vi "Periodic Tasks.vi"(8 "error in":errorcluster) -> ()   [LabVIEW 2014]
doc: "This VI runs in parallel to other tasks. It can contain as many user-defined periodic loops as you need. These can carry out PID or other sorts of timed response."
uses:
  1756_Code/General_VI/Global Var.vi
  <vilib>/Rock Robotics/Network Tables/SD Write Numeric Array.vi
panel:
  out "output cluster":T1
  in  "Num_Avg":dbl=10.0
  out "Autro":T2
  out "Master_Auto_Stop_Value":bool
  out "Auto_State":dbl(graph)
  in  "Reset_Enable":bool
  out "Compressor Running":bool
  out "Compressor Monitoring":bool
  out "Yaw":dbl
  out "Yaw":cluster{dbl, dbl}(knob)={0.0, 152.0639793131716} scale=-180.0..180.0
  out "Z Ang":dbl(graph)
  out "FreeFall":bool
  out "Motion":bool
  out "Anomaly":bool
  out "R/P Alpha":dbl
  out "Yaw Alpha":dbl
  in  "tau acc (s)":dbl=0.047 format="%#_13g"
  in  "tau mag (s)":dbl=0.06 format="%#_13g"
  in  "Tilt Comp (Yaw)":bool
  # "FRC Team 836, The RoboBees: Sensor Fusion Demonstration / Designed for roboRIO\nDescription:\nThis series of Inertial Measurement Unit (IMU) subVIs is patterened after the WPI series for reading sensors, and includes several\nadditional IMU Application subVIs.  These application subVIs do the math required for sensor fusion, forming a basic Attitude\nand Heading Reference System (AHRS), with drift-free Roll, Pitch and Yaw outputs.  An IMU typically consists of a 3-axis \nAccelerometer, Rate Gyroscope, and Magnetometer (sometimes the Mag is absent, resulting in reduced capability).  Although\ntechnically incorrect, these devices are often referred to as 9 Degrees-of-Freedom (DoF) sensors (3 sensors with each 3\naxes in XYZ = 9 DoF). \n\nCompatible IMUs:\nThese IMU subVIs are designed to be used with the Adafruit 9-DoF IMU Breakout - containing L3GD20 (Gyro) + LSM303 \n(Accelerometer and Magnetometer) chips (Product ID: 1714), or the Adafruit 10-DoF IMU Breakout - whichs adds the BMP180\nchip (Product ID: 1604).  The 10-DoF IMU adds a Barometer for air temperature and pressure measurements (for indicating\naltitude, not attitude), and is not currently implemented.  The two IMU Application subVIs, COMPLE FILTER and TILT, are\nagnostic of IMU model, and compatible with separate sensors, as long as all sensor axes are aligned properly."
  # "AdaFruit 1714"
  # "Sensor Orientation:\nWhen Sensor oriented with positive X-axis\npointing forward, and positive Y-axis\npointing left, and positive Z axis pointing up :\n\nRoll is rotation about X-axis, clockwise roll,\n(looking in + X direction), is positive.\n\nPitch is rotation about Y-axis, clockwise pitch\n(looking in + Y direction), is positive.\n\nYaw is rotation about Z-axis, clockwise yaw\n(looking in + Z direction), is positive."
  # "Robot\nFront"
  # "RoboBees IMU and AHRS Demo Instructions:\n(1) Connect IMU to I2C port (4 wires: 5v/Gnd/SDA/SCK) on roboRIO.\n      Secure the IMU on Robot, orient as described at right.\n(2) Change the IP address of the roboRIO in the RoboBees IMU Demo project.\nYou can do this by right-clicking on RT CompactRIO Target in the project, selecting\nProperties, and modifying the IP Address setting in the General Category to match\nthat of your roboRIO.\n(3) Open Front Panel of the IMU OPEN subVI, you'll need that for step 8.\n(4) Establish Comm and Run this program (use Run Button deploy, not Build and deploy).\n(5) Follow the dialog boxes to perform Magnetometer Calibration.\n(6) Upon cal completion, observe Roll, Pitch, Yaw gauges as you (re)orient your sensor/robot.\n(7) Observe the 9 DoF display graphs for Gyro, Accel, and Mag in each XYZ axes.  The graphs are\n       useful in understanding how the sensors respond, but it's best to disable them once you no\n       longer need them, as they slow the dynamic response of the code under a Run button\n       deploy.  A simple way to do this is to wrap a Diagram Disable Structure (Structures Menu)\n       around the chart indicators on the Block Diagram. \n(8) Observe result of Magnetometer cal graph on the IMU OPEN front panel.  Use adjacent\n      graph display for reference.\n(9) If you don't like Mag cal result, repeat Mag cal by rerunning program.  See comments\nin IMU OPEN code for guidance.  If cal ok, stop program and load the 4 Mag cal\nparameters displayed in IMU OPEN (two each for X and Y axes), into Mag Set Cluster just below.\n(10) Set MagCal switch to false, then rerun this program.  This config is for competition.\n(11) Adjust the Loop Period as desired.  See implementation notes in IMU READ VI for guidance.\n(12) Adjust the Accelerometer tau and Magnetometer tau values as desired.  See implementation\n       notes in COMPLE FILTER VI  for guidance.\n(13) The Gyro/Accel cal process w/in IMU OPEN will auto-recal if it detects excessive\n        variation in the sample dataset, which likely indicates robot was bumped during cal.\n        Gently shake robot during program startup and observe BadCal indicators.\n(14) The roboRIO has two seperate I2C buses, On-Board and MXP.  This code works with the\n        On-Board I2C bus, but currently throws an error on the MXP I2C bus, tested with a Rev\n        Robotics expansion board.  \n\nPls provide attribution to FRC Team 836, The RoboBees if you find this useful !!"
  # "roboRIO I2C    DIO-0  V     Gnd    SCL     SDA"
  # "Sensor Fusion Design:"
  # "Note that Period (dt) can probably be reduced to less than 20 ms before Timed Loop starts running late, in this demo, since it's the only code running.  Using these IMU VIs in your code, however, may require a longer loop period to allow the CPU time to execute your other robot code  - you can use the same technique of adjusting the period while monitoring the Late indicator for optimization when you integrate these VIs into your code.  You can disable the 9 DoF graphs to considerably improve speed of code (when deployed with the Run button), in which case Period can be much lower (~3 ms, again, provided this is the only code running).  Benchmark was against 2015 roboRIO."
  # "Sensor Fusion Settings"
  # "Adjust these tau settings to optimize the sensor fusion.  tau acc affects\nRoll and Pitch.  tau mag affects Yaw.   Consider that alpha = tau / (tau + dt),\nand that alpha is what affects the fusion performance.  An alpha of about 0.7 for\nRoll and Pitch, and an alpha of about 0.6 for Yaw appear to be good starting points."
  # "Enabling this corrects Yaw error when Pitch and Roll are\nnon-zero, however, Yaw will be affected by Accelerometer\nmovement and noise.  Reference IMU Comple Filter subVI\nnotes for more insight on this tradeoff."
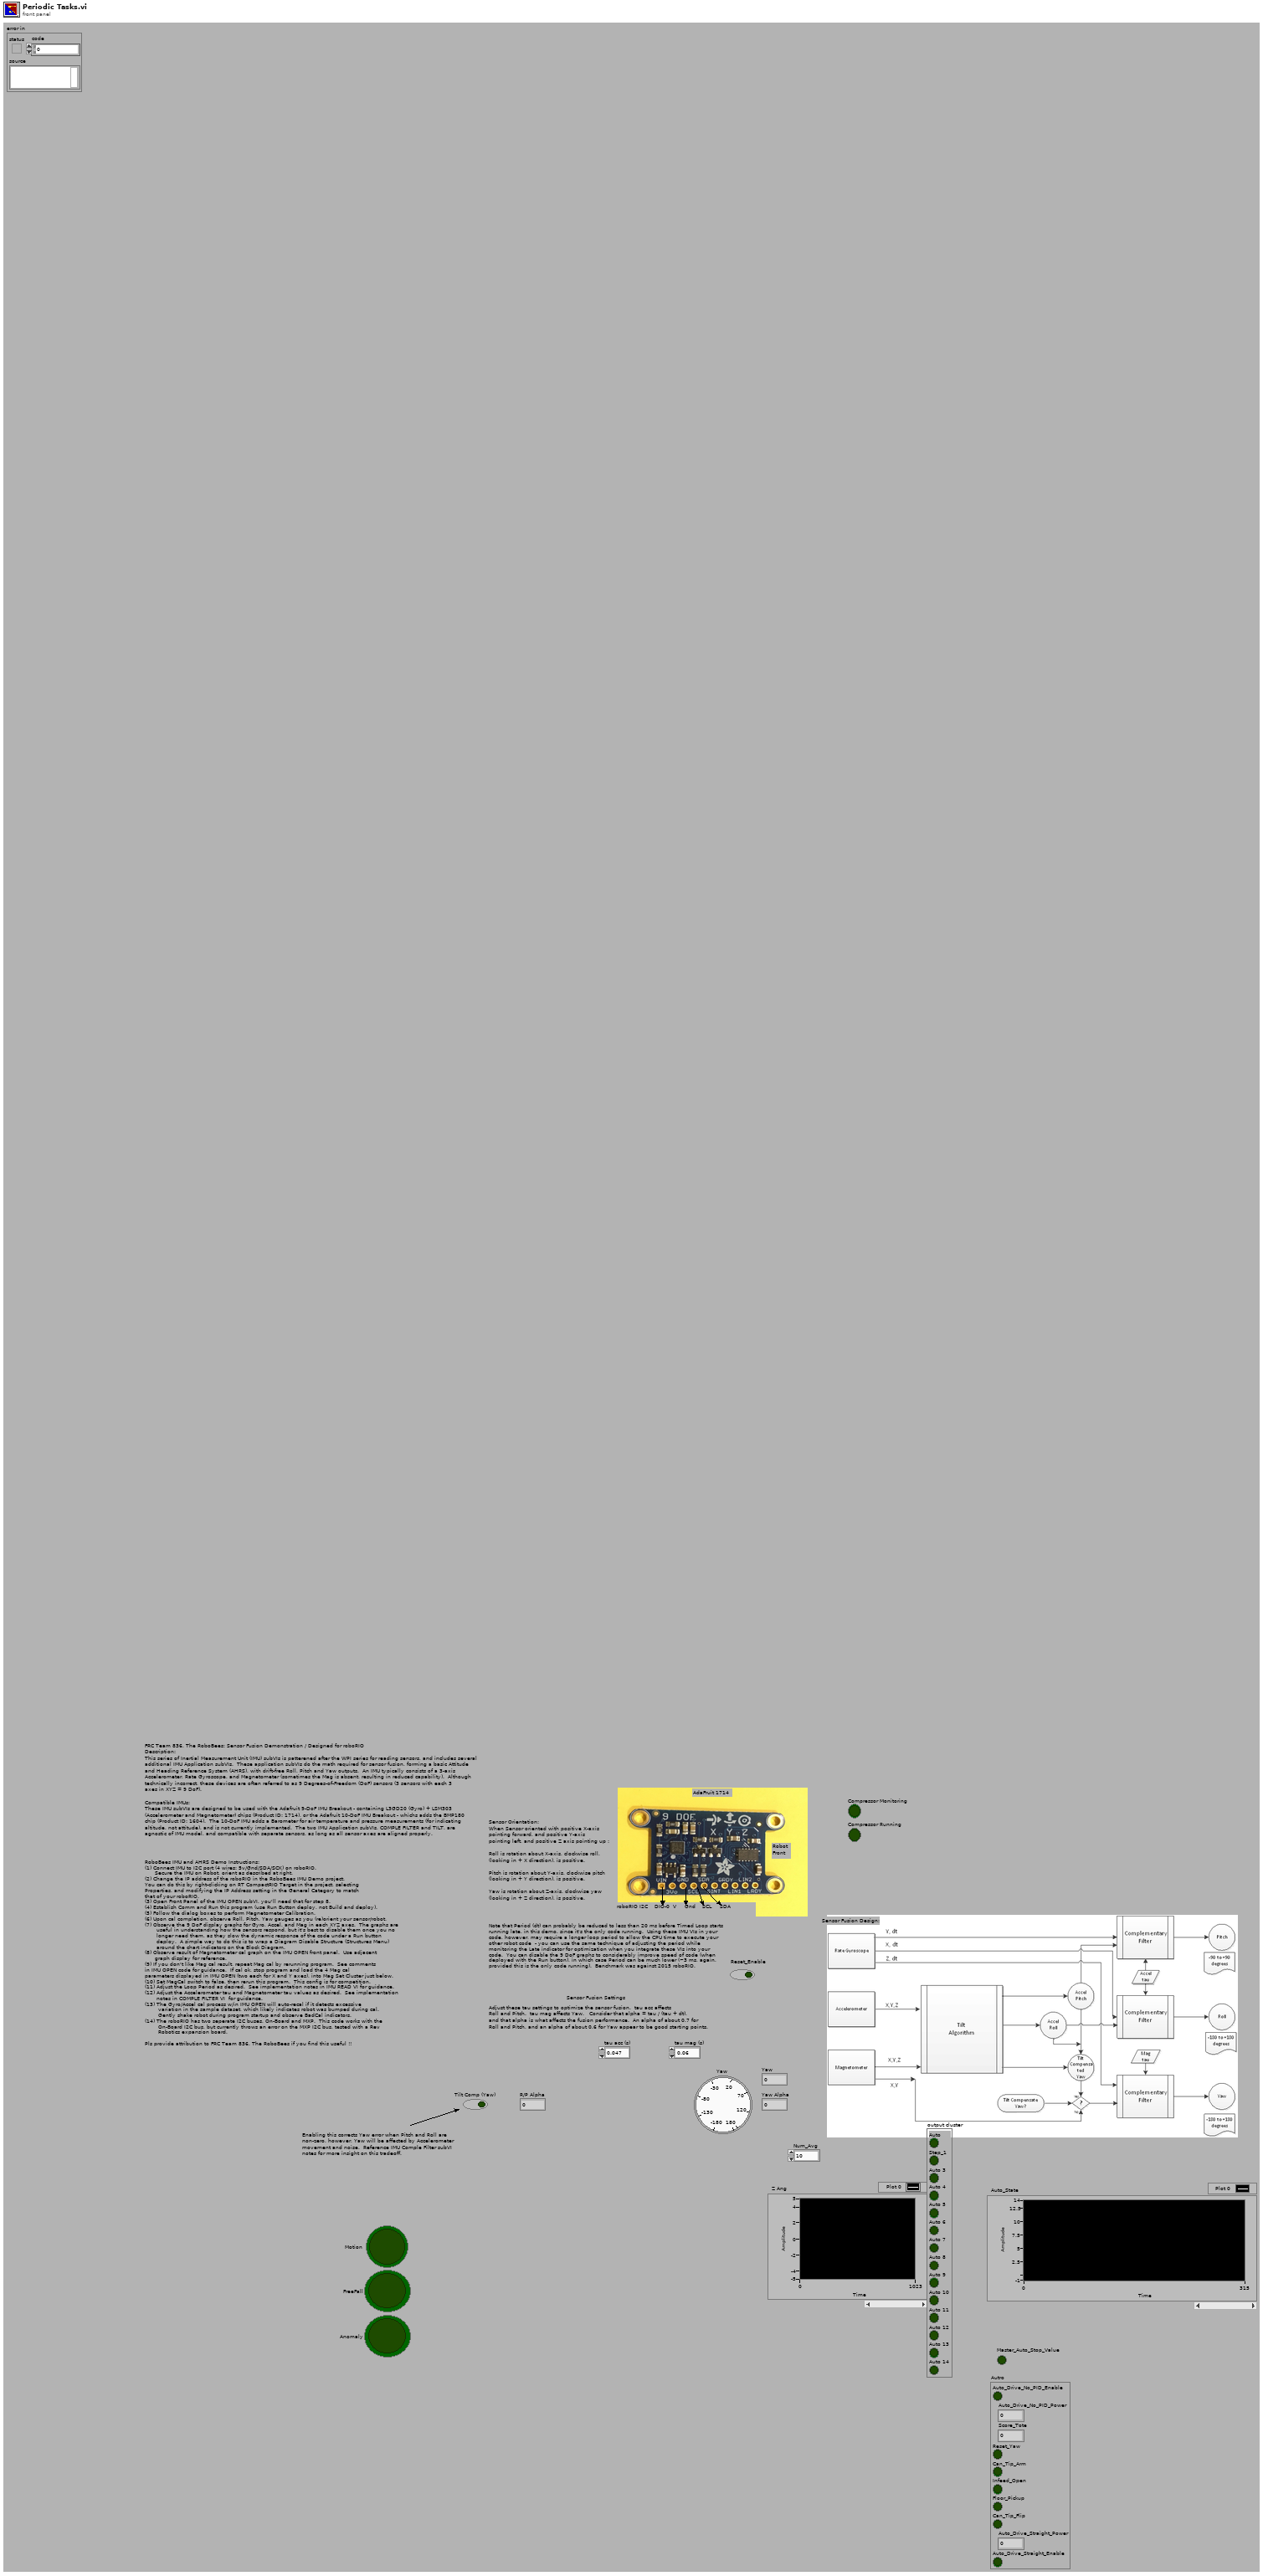
[diagram p1: front panel]
types:
  T1 = cluster{"Auto":bool, "Step_1":bool, "Auto 3":bool, "Auto 4":bool, "Auto 5":bool, "Auto 6":bool, "Auto 7":bool, "Auto 8":bool, "Auto 9":bool, "Auto 10":bool, "Auto 11":bool, "Auto 12":bool, "Auto 13":bool, "Auto 14":bool}
  T2 = cluster{"Auto_Drive_No_PID_Enable":bool, "Auto_Drive_No_PID_Power":dbl, "Score_Tote":dbl, "Reset_Yaw":bool, "Can_Tip_Arm":bool, "Infeed_Open":bool, "Floor_Pickup":bool, "Can_Tip_Flip":bool, "Auto_Drive_Straight_Power":dbl, "Auto_Drive_Straight_Enable":bool}
  T3 = typedef "WPI_JoystickDevRef.ctl" = cluster{"Device":T4}
  T4 = typedef "WPI_JoystickDeviceEnum.ctl" = enum16{"USB 0", "USB 1", "USB 2", "USB 3", "USB 4", "USB 5"}
  T5 = typedef "WPI_RobotDriveDevRef.ctl" = cluster{"DevStatus":errorcluster, "Motors[]":T6[], "Square Inputs":bool, "Max Output":dbl}
  T6 = typedef "WPI_MotorControlDeviceRef.ctl" = cluster{"DeviceStatus":errorcluster, "Type":T7, "PWM":cluster{"Controller":T8, "PWM Channel":T9, "DeadBand":T10}, "CAN":cluster{"Device Number":u8, "Control Mode":T11, "Semaphore":T12, "Max Vout":dbl, "TalonSRX Control Mode":T13}, "Invert":bool, "TransformRef":T14, "InvTransformRef":T14}
  T7 = typedef "WPI_MotorControlType.ctl" = enum16{"PWM", "CAN", "CANTalonSRX"}
  T8 = typedef "FPGA_TypedefDigitalModule.ctl" = enum16{"Controller 1"}
  T9 = typedef "FPGA_DIOPWMChannel.ctl" = enum8{"PWM 0", "PWM 1", "PWM 2", "PWM 3", "PWM 4", "PWM 5", "PWM 6", "PWM 7", "PWM 8", "PWM 9", "PWM MXP 0", "PWM MXP 1", "PWM MXP 2", "PWM MXP 3", "PWM MXP 4", "PWM MXP 5", "PWM MXP 6", "PWM MXP 7", "PWM MXP 8", "PWM MXP 9", "Invalid"}
  T10 = typedef "WPI_PWMDeadband.ctl" = cluster{"Name":string, "maxPositivePwm":i32, "minPositivePwm":i32, "centerPwm":i32, "maxNegativePwm":i32, "minNegativePwm":i32, "angularRange":u16}
  T11 = typedef "WPI_CANJaguar_ControlMode.ctl" = enum8{"Percent VBus", "Current", "Speed", "Position", "Voltage"}
  T12 = typedef "Semaphore RefNum" = refnum<k1>
  T13 = typedef "WPI_CANTalonSRX_APIControlMode.ctl" = enum8{"Percent VBus", "Speed", "Position", "Slave", "Unchanged / Invalid"}
  T14 = typedef "WPI_PWMTransform_ConPane.ctl" = refnum<vi>
  T15 = typedef "WPI_EncoderDevRef.ctl" = cluster{"DevStatus":errorcluster, "EncoderIndex":T16, "CounterIndex":T17, "DistancePerCount":dbl, "Decoding Type":T18}
  T16 = typedef "FPGA_EncoderIdx.ctl" = enum8{"Enc 0", "Enc 1", "Enc 2", "Enc 3", "Enc 4", "Enc 5", "Enc 6", "Enc 7", "Invalid"}
  T17 = typedef "FPGA_CounterCtrSystemIndex.ctl" = enum8{"Ctr 0", "Ctr 1", "Ctr 2", "Ctr 3", "Ctr 4", "Ctr 5", "Ctr 6", "Ctr 7", "Invalid"}
  T18 = typedef "WPI_EncoderType.ctl" = enum16{"1x", "2x", "4x"}
  T19 = typedef "WPI_SwitchDevRef.ctl" = cluster{"DevStatus":errorcluster, "DIO Channel":T20, "Controller":T8, "CntIndex":T17, "Normally Closed":bool}
  T20 = typedef "FPGA_DIOChannel.ctl" = enum8{"DIO 0", "DIO 1", "DIO 2", "DIO 3", "DIO 4", "DIO 5", "DIO 6", "DIO 7", "DIO 8", "DIO 9", "DIO MXP 0", "DIO MXP 1", "DIO MXP 2", "DIO MXP 3", "DIO MXP 4", "DIO MXP 5", "DIO MXP 6", "DIO MXP 7", "DIO MXP 8", "DIO MXP 9", "DIO MXP 10", "DIO MXP 11", "DIO MXP 12", "DIO MXP 13", "DIO MXP 14", "DIO MXP 15", "Invalid"}
  T21 = typedef "WPI_AnalogChannelDevRef.ctl" = cluster{"DevStatus":errorcluster, "Controller":T22, "Analog Channel":T23}
  T22 = typedef "FPGA_TypedefAnalogModule.ctl" = enum16{"Controller 1"}
  T23 = typedef "FPGA_AIChannel.ctl" = enum8{"AI 0", "AI 1", "AI 2", "AI 3", "AI MXP 0", "AI MXP 1", "AI MXP 2", "AI MXP 3", "Invalid"}
  T24 = typedef "IMUDevRef.ctl" = cluster{"DevStatus":errorcluster, "Gyro Address":u8, "Gyro Range":u8, "Mean Rates":cluster{"Xmo":dbl, "Ymo":dbl, "Zmo":dbl}, "StdDev Rates":cluster{"Xsdo":dbl, "Ysdo":dbl, "Zsdo":dbl}, "Fast":bool, "Reset":bool, "Accel Address":u8, "Accel Range":u8, "Accel Scale":cluster{"Xscale":dbl, "Yscale":dbl, "Zscale":dbl}, "Mag Address":u8, "Mag Range":u8, "G Sense":bool, "A Sense":bool, "M Sense":bool, "Accel Offset":cluster{"Xzero":dbl, "Yzero":dbl, "Zzero":dbl}, "Motion Thresh":dbl, "Mag Scale":cluster{"Xscale":dbl, "Yscale":dbl, "Zscale":dbl}, "Mag Offset":cluster{"Xzero":dbl, "Yzero":dbl, "Zzero":dbl}, "I2C Bus":T25, "Handle":i32, "Controller":T8, "Anomaly Thresh":dbl, "Local Mag":dbl}
  T25 = typedef "i2c_bus.ctl" = enum16{"I2C On-Board", "I2C MXP", "Invalid"}
  T26 = typedef "WPI_CompressorDevRef.ctl" = cluster{"DevStatus":errorcluster, "Pneumatics Control Module":u8}
  T27 = typedef "WPI_SolenoidDevRef.ctl" = cluster{"DevStatus":errorcluster, "Pneumatics Control Module":u8, "Forward Solenoid Channel":T28, "Reverse Solenoid Channel":T28}
  T28 = typedef "WPI_SolenoidChannel.ctl" = enum8{"Solenoid 0", "Solenoid 1", "Solenoid 2", "Solenoid 3", "Solenoid 4", "Solenoid 5", "Solenoid 6", "Solenoid 7", "Invalid"}
  T29 = cluster{"Joystick":cluster{"Drive_Joystick":T3, "Imp_Joystick":T3}, "Motor":cluster{"Left and Right Motors":T5, "Left_Intake":T6, "Right_Intake":T6, "Elevator_Lift":T6, "Elevator_Arm_Left":T6, "Elevator_Arm_Right":T6}, "Encoder":cluster{"Left_Drive_Speed":T15, "Auto_2_Tote":T19, "Auto_Cans":T19, "Auto_Cans_Delay":T19}, "Analog":cluster{"Tote_Detect_1":T21, "Tote_Detect_2":T21, "Ele_Pos_Yoyo":T21, "Auto_Switch":T21}, "IMU_Reft_Num":T24, "Pneumatics":cluster{"Compressor":T26, "Arm_Sol":T27, "Infeed_Pneu":T27, "Can_Tip_Flip":T27, "Can_Tip_Arm":T27, "Can_Door_Arm":T27, "Arm_Sol_Ext":T27}}
  T30 = cluster{"Store_Auto":bool, "Exit_Auto":bool, "Infeed cmd":dbl, "Store_Auto_High":bool}
  T31 = cluster{"Station_Auto":bool, "Pickup_2_Auto":bool, "Infeed_cmd":dbl, "Open_Infeed":bool}
  T32 = cluster{"Open_Infeed":bool, " Raise_to_Step":bool, "Step 1":bool, "Step_3":bool}
  T33 = cluster{"Global_Var":cluster{"Eject":dbl, "Eject_Manual":dbl, " Station_Pickup":bool, "Arm_Pos":bool, "Elevator":dbl, "Exit_Pos":bool, "Floor_Pickup":bool, "Reset_Yaw":bool, "Step_Pos":bool, "Store_Pos":bool, "Yaw":dbl, "Score_Tote":bool, "Score_Step":bool, "Carry":bool, "Step_3":bool, "Infeed_Open":bool, "Can_Tip_Arm":bool, "Can_Tip_Flip":bool, "Step_1":bool, "Can_Door":bool, "Store_High":bool}, "Sensor_Val":cluster{"Left_Drive_Distance":dbl, "Tote_Detect_1":bool, "Tote_Detect_2":bool, "Ele_Pos_Yoyo":dbl, "Ele_At_Pos in":bool}}
  T34 = cluster{"Eject":dbl, "Eject_Manual":dbl, " Station_Pickup":bool, "Arm_Pos":bool, "Elevator":dbl, "Exit_Pos":bool, "Floor_Pickup":bool, "Reset_Yaw":bool, "Step_Pos":bool, "Store_Pos":bool, "Yaw":dbl, "Score_Tote":bool, "Score_Step":bool, "Carry":bool, "Step_3":bool, "Infeed_Open":bool, "Can_Tip_Arm":bool, "Can_Tip_Flip":bool, "Step_1":bool, "Can_Door":bool, "Store_High":bool}
  T35 = cluster{"Left_Drive_Distance":dbl, "Tote_Detect_1":bool, "Tote_Detect_2":bool, "Ele_Pos_Yoyo":dbl, "Ele_At_Pos in":bool}
  T36 = cluster{"Global_Var":cluster{"Eject":dbl, "Eject_Manual":dbl, " Station_Pickup":bool, "Arm_Pos":bool, "Elevator":dbl, "Exit_Pos":bool, "Floor_Pickup":bool, "Reset_Yaw":bool, "Step_Pos":bool, "Store_Pos":bool, "Yaw":dbl, "Score_Tote":bool, "Score_Step":bool, "Carry":bool, "Step_3":bool, "Infeed_Open":bool, "Can_Tip_Arm":bool, "Can_Tip_Flip":bool, "Step_1":bool, "Can_Door":bool, "Store_High":bool}, "Sensor_Val":cluster{"Left_Drive_Distance":dbl, "Tote_Detect_1":bool, "Tote_Detect_2":bool, "Ele_Pos_Yoyo":dbl, "Ele_At_Pos in":bool}, "Floor":cluster{"Store_Auto":bool, "Exit_Auto":bool, "Infeed cmd":dbl, "Store_Auto_High":bool}, "Station":cluster{"Station_Auto":bool, "Pickup_2_Auto":bool, "Infeed_cmd":dbl, "Open_Infeed":bool}, "Score_Tote":cluster{"Lower to Exit":bool, "Open Arms":bool}, "Score_Step":cluster{"Open_Infeed":bool, " Raise_to_Step":bool, "Step 1":bool, "Step_3":bool}, "Carry_Auto":cluster{"Lower to Carry":bool, "Open Arms":bool}}
  T37 = cluster{"Global_Var":cluster{"Eject":dbl, "Eject_Manual":dbl, " Station_Pickup":bool, "Arm_Pos":bool, "Elevator":dbl, "Exit_Pos":bool, "Floor_Pickup":bool, "Reset_Yaw":bool, "Step_Pos":bool, "Store_Pos":bool, "Yaw":dbl, "Score_Tote":bool, "Score_Step":bool, "Carry":bool, "Step_3":bool, "Infeed_Open":bool, "Can_Tip_Arm":bool, "Can_Tip_Flip":bool, "Step_1":bool, "Can_Door":bool, "Store_High":bool}, "Sensor_Val":cluster{"Left_Drive_Distance":dbl, "Tote_Detect_1":bool, "Tote_Detect_2":bool, "Ele_Pos_Yoyo":dbl, "Ele_At_Pos in":bool}, "Floor":cluster{"Store_Auto":bool, "Exit_Auto":bool, "Infeed cmd":dbl, "Store_Auto_High":bool}, "Station":cluster{"Station_Auto":bool, "Pickup_2_Auto":bool, "Infeed_cmd":dbl, "Open_Infeed":bool}, "Score_Tote":cluster{"Lower to Exit":bool, "Open Arms":bool}, "Score_Step":cluster{"Open_Infeed":bool, " Raise_to_Step":bool, "Step 1":bool, "Step_3":bool}, "Carry_Auto":cluster{"Lower to Carry":bool, "Open Arms":bool}, "Pos_Arb":cluster{"Pos_Des":dbl, "Pos_Active":bool}}
  T38 = typedef "Gyro.ctl" = cluster{"Xrate":dbl, "Yrate":dbl, "Zrate":dbl, "Xdeg":dbl, "Ydeg":dbl, "Zdeg":dbl, "dt":dbl}
  T39 = typedef "Accel.ctl" = cluster{"Xaccel":dbl, "Yaccel":dbl, "Zaccel":dbl, "Motion":bool, "Threshold":dbl, "FreeFall":bool}
  T40 = typedef "Mag.ctl" = cluster{"Xmag":dbl, "Ymag":dbl, "Zmag":dbl, "Anomaly":bool}
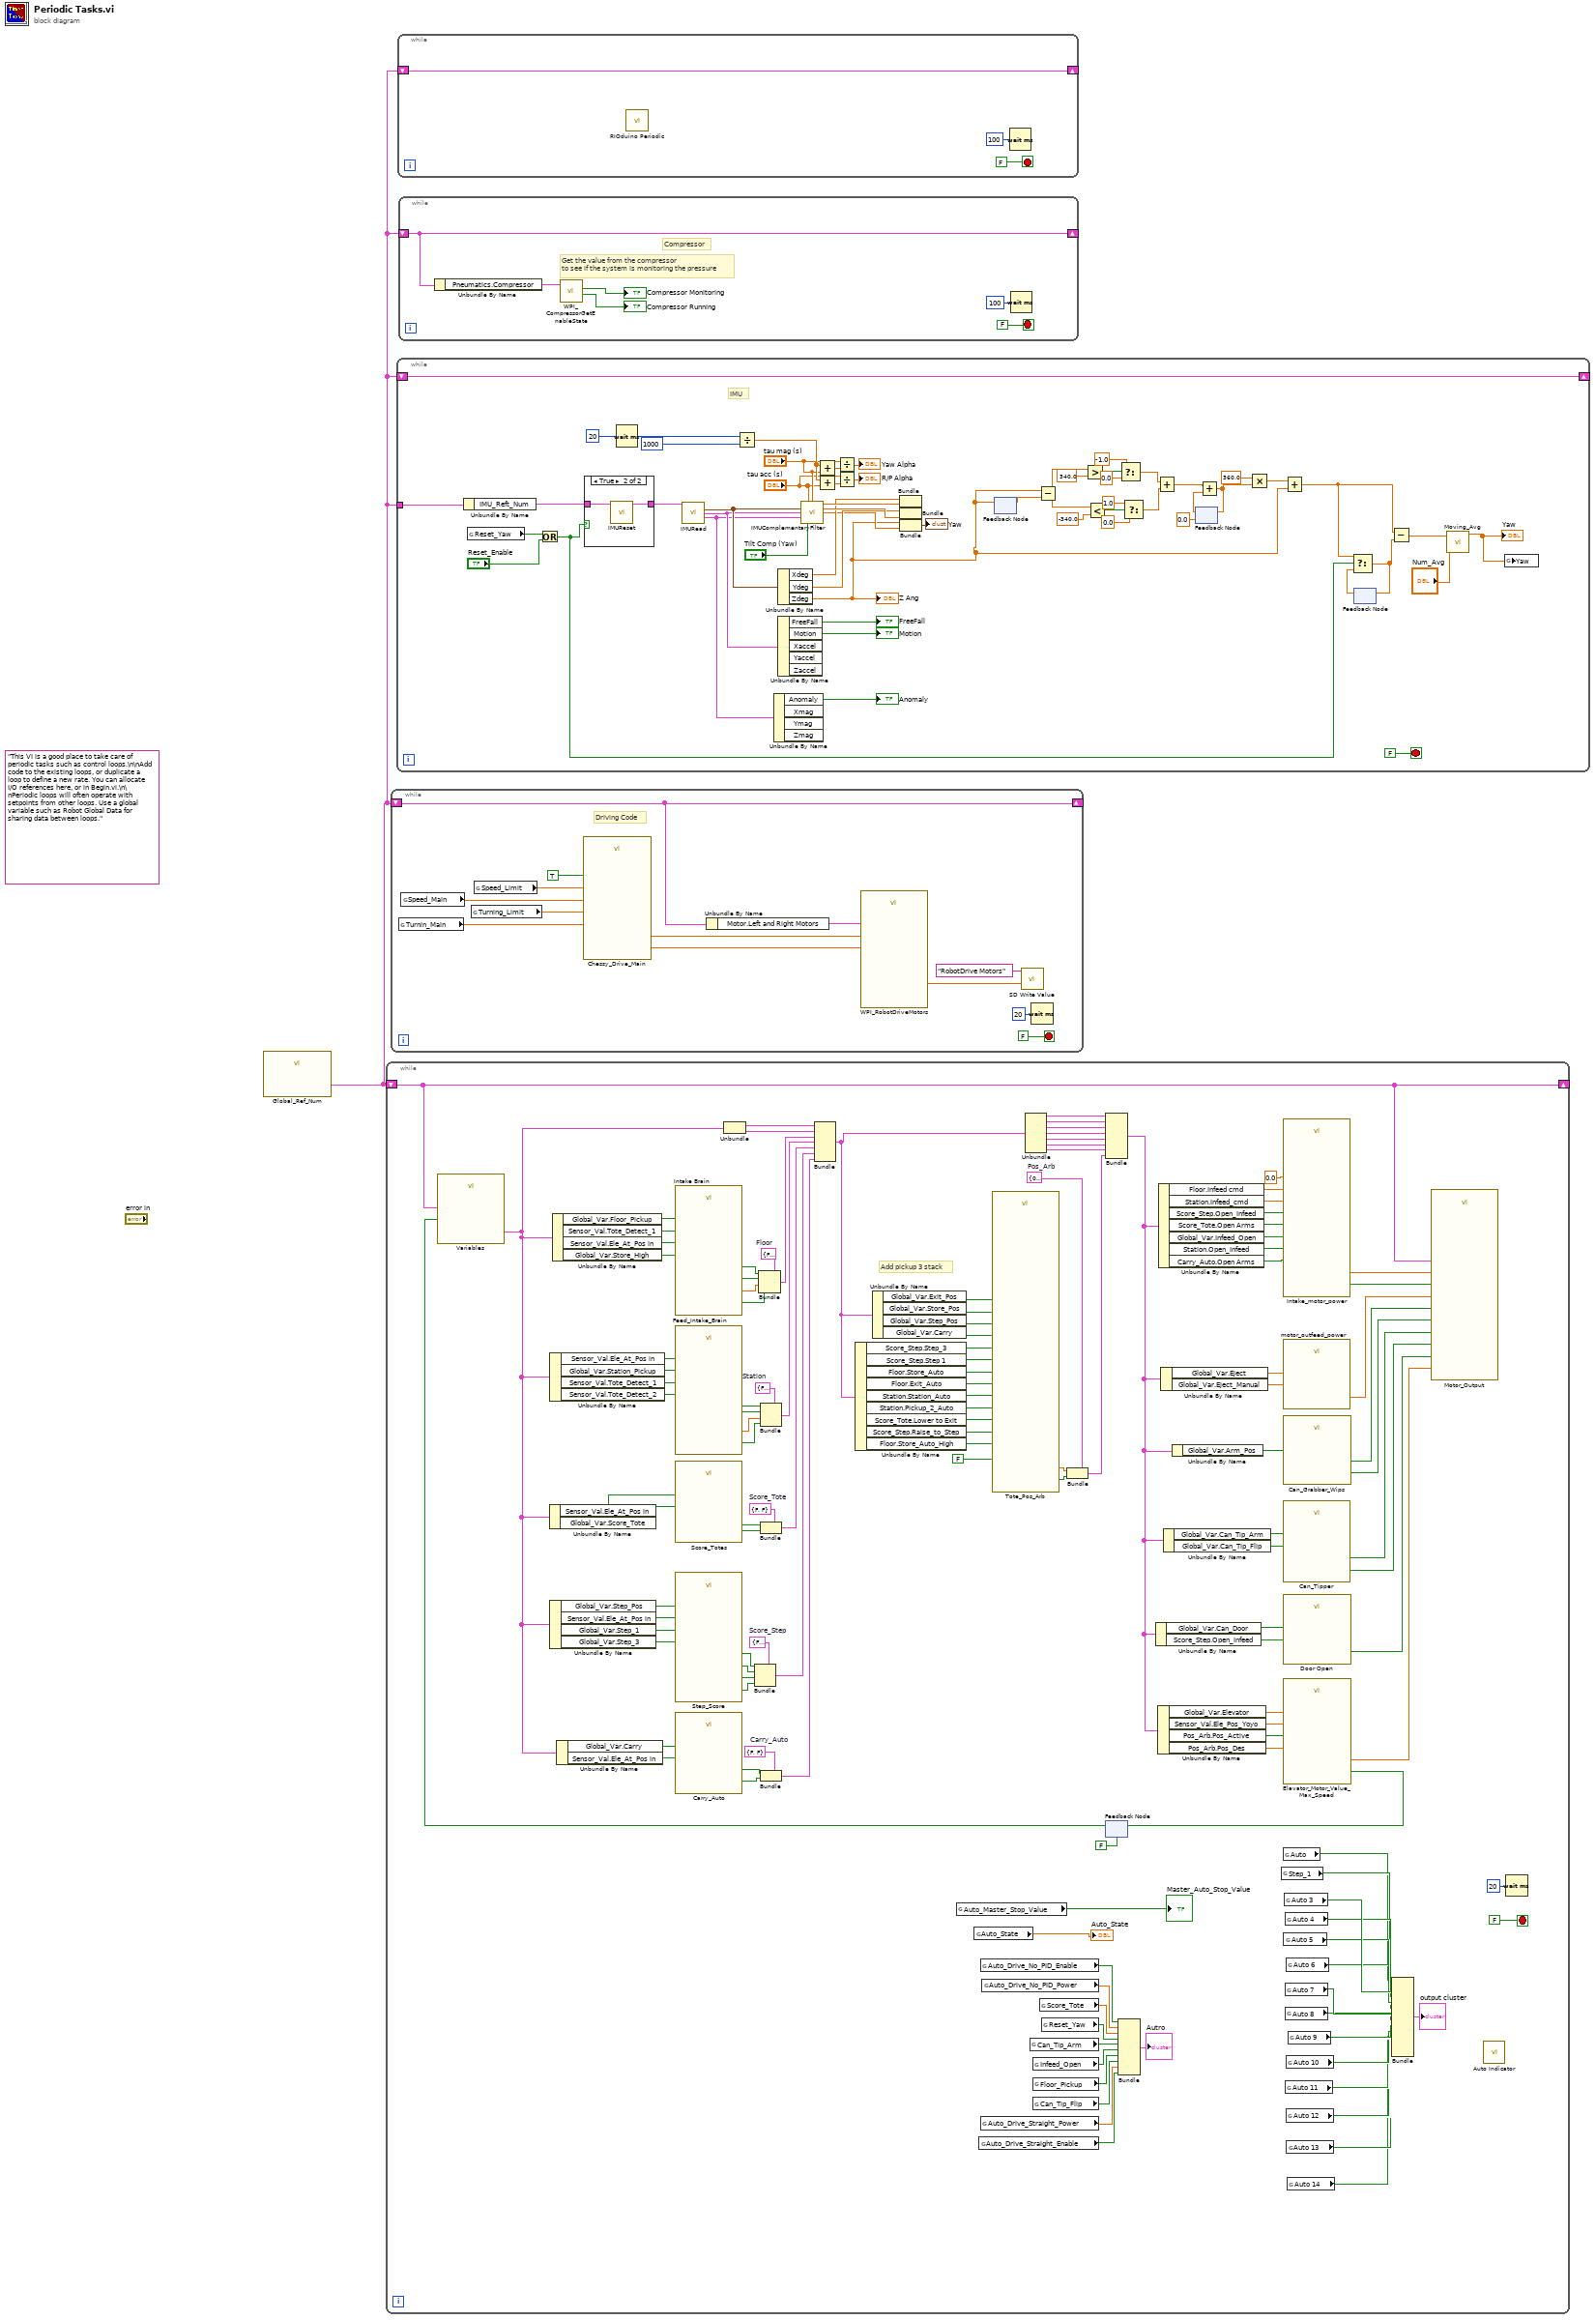
[diagram p0: block diagram]
diagram:
  (unwired) "This VI is a good place to take care of periodic tasks such as control loops.\n\nAdd code to the existing loops, or duplicate a loop to define a new rate. You can allocate I/O references here, or in Begin.vi.\n\nPeriodic loops will often operate with setpoints from other loops. Use a global variable such as Robot Global Data for sharing data between loops."
  n1 = call "Global_Ref_Num.vi"() -> ("Ref_Num"=w1:T29)  [unwired: 10 in]
  n2 = while {
    shift-right: [w11] -> _
    shift-left: w1 -> [w11]
    stop <- FALSE stop-if-true
    w14 = T30 {"Store_Auto"=FALSE, "Exit_Auto"=FALSE, "Infeed cmd"=0.0, "Store_Auto_High"=FALSE}  # Floor
    w52 = cluster{"Lower to Carry":bool, "Open Arms":bool} {"Lower to Carry"=FALSE, "Open Arms"=FALSE}  # Carry_Auto
    w62 = T31 {"Station_Auto"=FALSE, "Pickup_2_Auto"=FALSE, "Infeed_cmd"=0.0, "Open_Infeed"=FALSE}  # Station
    w68 = T32 {"Open_Infeed"=FALSE, " Raise_to_Step"=FALSE, "Step 1"=FALSE, "Step_3"=FALSE}  # Score_Step
    w77 = cluster{"Pos_Des":dbl, "Pos_Active":bool} {"Pos_Des"=0.0, "Pos_Active"=FALSE}  # Pos_Arb
    w78 = cluster{"Lower to Exit":bool, "Open Arms":bool} {"Lower to Exit"=FALSE, "Open Arms"=FALSE}  # Score_Tote
    # "Add pickup 3 stack"
    n3 = global read "Global Var.vi" "Auto_Master_Stop_Value"() -> (→"Master_Auto_Stop_Value":bool)
    n4 = global read "Global Var.vi" "Auto_State"() -> (→"Auto_State":dbl)
    n5 = global read "Global Var.vi" "Auto_Drive_Straight_Enable"() -> (w37:bool)
    n6 = global read "Global Var.vi" "Auto_Drive_No_PID_Enable"() -> (w46:bool)
    n7 = global read "Global Var.vi" "Auto_Drive_Straight_Power"() -> (w38:dbl)
    n8 = global read "Global Var.vi" "Auto_Drive_No_PID_Power"() -> (w45:dbl)
    n9 = global read "Global Var.vi" "Can_Tip_Arm"() -> (w42:bool)
    n10 = global read "Global Var.vi" "Infeed_Open"() -> (w41:bool)
    n11 = global read "Global Var.vi" "Floor_Pickup"() -> (w40:bool)
    n12 = global read "Global Var.vi" "Can_Tip_Flip"() -> (w39:bool)
    n13 = global read "Global Var.vi" "Score_Tote"() -> (w44:dbl)
    n14 = global read "Global Var.vi" "Reset_Yaw"() -> (w43:bool)
    n15 = feedback #1(FALSE ("Pos_Check")) -> (w132:bool)
    n16 = call "Variables.vi"("Ele_At_Pos"=w132, "Ref_Num"=w11) -> ("Var"=w57:T33)  [unwired: 9 in]
    n17 = Unbundle By Name(w57) -> ("Sensor_Val.Ele_At_Pos in"=w100:bool, "Global_Var.Score_Tote"=w91:bool)
    n18 = Unbundle By Name(w57) -> ("Sensor_Val.Ele_At_Pos in"=w130:bool, "Global_Var.Station_Pickup"=w129:bool, "Sensor_Val.Tote_Detect_1"=w128:bool, "Sensor_Val.Tote_Detect_2"=w127:bool)
    n19 = Unbundle By Name(w57) -> ("Global_Var.Step_Pos"=w90:bool, "Sensor_Val.Ele_At_Pos in"=w89:bool, "Global_Var.Step_1"=w67:bool, "Global_Var.Step_3"=w66:bool)
    n20 = Unbundle By Name(w57) -> ("Global_Var.Floor_Pickup"=w131:bool, "Sensor_Val.Tote_Detect_1"=w102:bool, "Sensor_Val.Ele_At_Pos in"=w103:bool, "Global_Var.Store_High"=w16:bool)
    n21 = Unbundle By Name(w57) -> ("Global_Var.Carry"=w56:bool, "Sensor_Val.Ele_At_Pos in"=w55:bool)
    n22 = call "Intake Brain.vi"("Floor_Pickup"=w131, "Ele_At_Pos"=w103, "Floor_Pickup_High"=w16, "Tote_Sensor_1"=w102) -> ("Exit_Auto"=w123:bool, "Store_Auto"=w122:bool, "Store_Auto_High"=w15:bool, "Infeed cmd"=w121:dbl)  [unwired: 4 in]
    n23 = call "Feed_Intake_Brain.vi"("Station_Pickup"=w129, "Ele_At_Pos"=w130, "Tote_Detect_2"=w127, "Tote_Detect_1"=w128) -> ("Open_Infeed"=w63:bool, "Infeed_cmd"=w124:dbl, "Pickup_2_Auto"=w125:bool, "Station_Auto"=w126:bool)  [unwired: 4 in]
    n24 = call "Score_Totes.vi"("Score_Tote"=w91, "Ele_At_Pos"=w100) -> ("Lower to Exit"=w99:bool, "Open Arms"=w98:bool)  [unwired: 8 in]
    n25 = call "Step_Score.vi"("Step_Score"=w90, "Step_3"=w66, "Step_1"=w67, "Ele_At_Pos"=w89) -> ("Step_3"=w69:bool, "Step 1"=w70:bool, "Raise_to_Step"=w71:bool, "Open_Infeed"=w72:bool)  [unwired: 4 in]
    n26 = call "Carry_Auto.vi"("Carry_Manual"=w56, "Ele_At_Pos"=w55) -> ("Lower to Carry"=w54:bool, "Open Arms"=w53:bool)  [unwired: 8 in]
    n27 = Unbundle(w57) -> ("Global_Var"=w116:T34, "Sensor_Val"=w115:T35)
    n28 = Bundle(cluster=w68, "Open_Infeed"=w72, "Raise_to_Step"=w71, "Step 1"=w70, "Step_3"=w69) -> (w95:T32)
    n29 = Bundle(cluster=w14, "Store_Auto"=w122, "Exit_Auto"=w123, "Infeed cmd"=w121, "Store_Auto_High"=w15) -> (w114:T30)
    n30 = Bundle(cluster=w62, "Station_Auto"=w126, "Pickup_2_Auto"=w125, "Infeed_cmd"=w124, "Open_Infeed"=w63) -> (w113:T31)
    n31 = Bundle(cluster=w78, "Lower to Exit"=w99, "Open Arms"=w98) -> (w97:cluster{"Lower to Exit":bool, "Open Arms":bool})
    n32 = Bundle(cluster=w52, "Lower to Carry"=w54, "Open Arms"=w53) -> (w51:cluster{"Lower to Carry":bool, "Open Arms":bool})
    n33 = Bundle("Global_Var"=w116, "Sensor_Val"=w115, "Floor"=w114, "Station"=w113, "Score_Tote"=w97, "Score_Step"=w95, "Carry_Auto"=w51) -> (w96:T36)  [unwired: 1 in]
    n34 = Unbundle By Name(w96) -> ("Score_Step.Step_3"=w65:bool, "Score_Step.Step 1"=w64:bool, "Floor.Store_Auto"=w120:bool, "Floor.Exit_Auto"=w119:bool, "Station.Station_Auto"=w112:bool, "Station.Pickup_2_Auto"=w111:bool, "Score_Tote.Lower to Exit"=w88:bool, "Score_Step.Raise_to_Step"=w87:bool, "Floor.Store_Auto_High"=w13:bool)
    n35 = Unbundle By Name(w96) -> ("Global_Var.Exit_Pos"=w83:bool, "Global_Var.Store_Pos"=w82:bool, "Global_Var.Step_Pos"=w81:bool, "Global_Var.Carry"=w80:bool)
    n36 = call "Tote_Pos_Arb.vi"("Ben"=FALSE, "Exit_Floor"=w119, "Exit"=w83, "Step"=w81, "Station_Station"=w112, "Store"=w82, "Store_Floor"=w120, "Pickup_2_Station"=w111, "Exit_Score"=w88, "Step_Step"=w87, "Carry"=w80, "Step_3"=w65, "Step_1"=w64, "Store High"=w13) -> ("Pos_Active"=w117:bool, "Pos_Des"=w118:dbl)  [unwired: 4 in]
    n37 = Unbundle(w96) -> ("Global_Var"=w94:T34, "Sensor_Val"=w110:T35, "Floor"=w109:T30, "Station"=w108:T31, "Score_Tote"=w93:cluster{"Lower to Exit":bool, "Open Arms":bool}, "Score_Step"=w92:T32, "Carry_Auto"=w50:cluster{"Lower to Carry":bool, "Open Arms":bool})
    n38 = Bundle(cluster=w77, "Pos_Des"=w118, "Pos_Active"=w117) -> (w49:cluster{"Pos_Des":dbl, "Pos_Active":bool})
    n39 = Bundle("Global_Var"=w94, "Sensor_Val"=w110, "Floor"=w109, "Station"=w108, "Score_Tote"=w93, "Score_Step"=w92, "Carry_Auto"=w50, "Pos_Arb"=w49) -> (w18:T37)  [unwired: 1 in]
    n40 = Bundle("Auto_Drive_No_PID_Enable"=w46, "Auto_Drive_No_PID_Power"=w45, "Score_Tote"=w44, "Reset_Yaw"=w43, "Can_Tip_Arm"=w42, "Infeed_Open"=w41, "Floor_Pickup"=w40, "Can_Tip_Flip"=w39, "Auto_Drive_Straight_Power"=w38, "Auto_Drive_Straight_Enable"=w37) -> (→"Autro":T2)  [unwired: 1 in]
    n41 = Unbundle By Name(w18) -> ("Global_Var.Can_Door"=w20:bool, "Score_Step.Open_Infeed"=w19:bool)
    n42 = Unbundle By Name(w18) -> ("Global_Var.Elevator"=w7:dbl, "Sensor_Val.Ele_Pos_Yoyo"=w6:dbl, "Pos_Arb.Pos_Active"=w5:bool, "Pos_Arb.Pos_Des"=w4:dbl)
    n43 = Unbundle By Name(w18) -> ("Floor.Infeed cmd"=w60:dbl, "Station.Infeed_cmd"=w107:dbl, "Score_Step.Open_Infeed"=w86:bool, "Score_Tote.Open Arms"=w85:bool, "Global_Var.Infeed_Open"=w79:bool, "Station.Open_Infeed"=w61:bool, "Carry_Auto.Open Arms"=w48:bool)
    n44 = Unbundle By Name(w18) -> ("Global_Var.Eject"=w106:dbl, "Global_Var.Eject_Manual"=w84:dbl)
    n45 = Unbundle By Name(w18) -> ("Global_Var.Can_Tip_Arm"=w76:bool, "Global_Var.Can_Tip_Flip"=w75:bool)
    n46 = Unbundle By Name(w18) -> ("Global_Var.Arm_Pos"=w8:bool)
    n47 = global read "Global Var.vi" "Step_1"() -> (w23:bool)
    n48 = call "Intake_motor_power.vi"("Open_Man"=w79, "Carry_Auto"=w48, "Open_Step"=w86, "Open_Station"=w61, "Open_Score"=w85, "Station_Infeed_cmd"=w107, "Infeed_Man_cmd"=0.0, "Floor_Infeed_cmd"=w60) -> ("Infeed_Pneu"=w101:bool, "Intake_Power"=w105:dbl)  [unwired: 2 in]
    n49 = call "motor_outfeed_power.vi"("Eject_Imp"=w84, "Eject_Driver"=w106) -> ("Ele_Outfeed_Power_Power"=w104:dbl)  [unwired: 9 in]
    n50 = call "Can_Tipper.vi"("Can_Tip_Flip"=w75, "Can_Tip_Arm"=w76) -> ("Can_Tip_Flip"=w73:bool, "Can_Tip_Arm"=w74:bool)  [unwired: 8 in]
    n51 = global read "Global Var.vi" "Auto"() -> (w22:bool)
    n52 = call "Can_Grabber_Wips.vi"("Trash can arm"=w8) -> ("Arm_Ext"=w9:bool, "Arm_Down"=w10:bool)  [unwired: 7 in]
    n53 = call "Door Open.vi"("Infeed Door In Auto"=w19, "Infeed Door In"=w20) -> ("Infeed Door Out"=w17:bool)  [unwired: 9 in]
    n54 = call "Elavator_Motor_Value_Max_Speed.vi"("Ele_Pos"=w6, "Pos_Des"=w4, "Pos_Active"=w5, "Ele_Manual"=w7) -> ("Ele_At_Pos"=w3:bool, "Ele_Lift_Power"=w2:dbl)  [unwired: 6 in]
    n55 = feedback-in #1(w3) -> ()
    n56 = global read "Global Var.vi" "Auto 5"() -> (w33:bool)
    n57 = global read "Global Var.vi" "Auto 3"() -> (w35:bool)
    n58 = global read "Global Var.vi" "Auto 4"() -> (w34:bool)
    n59 = global read "Global Var.vi" "Auto 7"() -> (w31:bool)
    n60 = global read "Global Var.vi" "Auto 8"() -> (w30:bool)
    n61 = global read "Global Var.vi" "Auto 11"() -> (w27:bool)
    n62 = global read "Global Var.vi" "Auto 6"() -> (w32:bool)
    n63 = global read "Global Var.vi" "Auto 10"() -> (w28:bool)
    n64 = global read "Global Var.vi" "Auto 12"() -> (w26:bool)
    n65 = global read "Global Var.vi" "Auto 13"() -> (w25:bool)
    n66 = global read "Global Var.vi" "Auto 14"() -> (w24:bool)
    n67 = global read "Global Var.vi" "Auto 9"() -> (w29:bool)
    n68 = Bundle("Auto"=w22, "Step_1"=w23, "Auto 3"=w35, "Auto 4"=w34, "Auto 5"=w33, "Auto 6"=w32, "Auto 7"=w31, "Auto 8"=w30, "Auto 9"=w29, "Auto 10"=w28, "Auto 11"=w27, "Auto 12"=w26, "Auto 13"=w25, "Auto 14"=w24) -> (→"output cluster":T1)  [unwired: 1 in]
    n69 = call "Motor_Output.vi"("Can_Door"=w17, "Ref_Num"=w11, "Can_Tip_Flip"=w73, "Can_Tip_Arm"=w74, "Infeed_Pneu"=w101, "Ele_Outfeed"=w104, "Arm_Sol_Pos"=w10, "Ele_Lift"=w2, "Intake"=w105, "Arm_Sol_Ext"=w9) -> ()  [unwired: 2 in]
    n70 = call "Auto Indicator.vi"() -> ()  [unwired: 12 in]
    n71 = Wait (ms)(milliseconds to wait=u32 20) -> ()  [unwired: 1 out]
  }
  n72 = while {
    shift-right: [w137] -> _
    shift-left: w1 -> [w137]
    stop <- FALSE stop-if-true
    # "Driving Code"
    n73 = global read "Global Var.vi" "Turnin_Main"() -> (w138:dbl)
    n74 = global read "Global Var.vi" "Speed_Main"() -> (w139:dbl)
    n75 = global read "Global Var.vi" "Turning_Limit"() -> (w140:dbl)
    n76 = global read "Global Var.vi" "Speed_Limit"() -> (w141:dbl)
    n77 = call "Chessy_Drive_Main.vi"("Speed_Main"=w139, "Turning_Main"=w138, "Speed_Limit"=w141, "Turning_Limit"=w140, "Quick_Turn"=TRUE) -> ("Left_Motor"=w145:dbl, "Right_Motor"=w144:dbl)  [unwired: 9 in]
    n78 = Unbundle By Name(w137) -> ("Motor.Left and Right Motors"=w136:T5)
    n79 = call <vilib>:"WPI_RobotDriveMotors.vi"("RightSpeed"=w144, "LeftSpeed"=w145, "RobotDriveDevRef"=w136) -> ("Motor Values"=w142:dbl[])  [unwired: 1 in, 7 out]
    n80 = call-poly <vilib>:"SD Write Value.vi"("Numeric Array"=w142, "Name"="RobotDrive Motors") -> ()  [unwired: 8 in, 2 out]
    n81 = Wait (ms)(milliseconds to wait=u32 20) -> ()  [unwired: 1 out]
  }
  n82 = while {
    shift-right: [w203] -> _
    shift-left: w1 -> [w203]
    tunnel: w1 -> [w202]
    stop <- FALSE stop-if-true
    # "IMU"
    n83 = Unbundle By Name(w202) -> ("IMU_Reft_Num"=w201:T24)
    n84 = global read "Global Var.vi" "Reset_Yaw"() -> (w175:bool)
    n85 = Or(x=w175, y="Reset_Enable") -> (x .or. y?=w173:bool)
    n86 = case shown="True" w173 {
      tunnel: w201 -> [w205 w207]
      tunnel: [w205 w206] -> w200
      frame False {
      }
      frame True {
        n87 = call "IMUReset.vi"("AdaIMUDevRef"=w207) -> ("AdaIMUDevRef Out"=w206:T24)  [unwired: 9 in, 1 out]
      }
    }
    n88 = Wait (ms)(milliseconds to wait=i64 20 ("Period (dt in ms)")) -> (millisecond timer value=w188:u32)
    n89 = call "IMURead.vi"("AdaIMUDevRef"=w200) -> ("Gyro"=w199:T38, "Accel"=w198:T39, "Mag"=w197:T40)  [unwired: 10 in, 2 out]
    n90 = Divide(x=w188, y=i64 1000) -> (x/y=w190:dbl)
    n91 = Unbundle By Name(w197) -> ("Anomaly"=→"Anomaly":bool)  [unwired: 3 out]
    n92 = Unbundle By Name(w199) -> ("Xdeg"=w180:dbl, "Ydeg"=w179:dbl, "Zdeg"=w149:dbl)
    "Z Ang" <- w149
    n93 = Unbundle By Name(w198) -> ("FreeFall"=→"FreeFall":bool, "Motion"=→"Motion":bool)  [unwired: 3 out]
    n94 = call "IMUComplementaryFilter.vi"("tau acc"="tau acc (s)", "tau mag"="tau mag (s)", "Gyro"=w199, "Accel"=w198, "Mag"=w197, "Tilt Comp (Yaw)"="Tilt Comp (Yaw)") -> ("Roll"=w182:dbl, "Pitch"=w181:dbl, "Yaw"=w151:dbl)  [unwired: 6 in, 1 out]
    n95 = Add(x=w190, y="tau mag (s)") -> (x+y=w194:dbl)
    n96 = Add(x=w190, y="tau acc (s)") -> (x+y=w192:dbl)
    n97 = Divide(x="tau mag (s)", y=w194) -> (x/y=→"Yaw Alpha":dbl)
    n98 = Divide(x="tau acc (s)", y=w192) -> (x/y=→"R/P Alpha":dbl)
    n99 = Bundle("Xdeg"=w180, "Roll"=w182) -> ()  [unwired: 1 in, 1 out]
    n100 = Bundle("Ydeg"=w179, "Pitch"=w181) -> ()  [unwired: 1 in, 1 out]
    n101 = Bundle("Zdeg"=w149, "Yaw"=w151) -> (→"Yaw":cluster{"Zdeg":dbl, "Yaw":dbl})  [unwired: 1 in]
    n102 = feedback-in #2(w149) -> ()
    n103 = feedback #2() -> (w169:dbl)  [unwired: 1 in]
    n104 = Subtract(x=w149, y=w169) -> (x-y=w167:dbl)
    n105 = Greater?(x=w167, y=340.0) -> (0:w165:bool)
    n106 = Less?(x=w167, y=-340.0) -> (x < y?=w162:bool)
    n107 = Select(t=-1.0, s=w165, f=0.0) -> (s? t:f=w159:dbl)
    n108 = Select(t=1.0, s=w162, f=0.0) -> (s? t:f=w158:dbl)
    n109 = Add(x=w159, y=w158) -> (x+y=w157:dbl)
    n110 = feedback #3(0.0) -> (w156:dbl)
    n111 = Add(x=w157, y=w156) -> (x+y=w154:dbl)
    n112 = feedback-in #3(w154) -> ()
    n113 = Multiply(x=360.0, y=w154) -> (x*y=w152:dbl)
    n114 = Add(x=w152, y=w149) -> (x+y=w150:dbl)
    n115 = feedback #4() -> (w176:dbl)  [unwired: 1 in]
    n116 = Select(t=w150, s=w173, f=w176) -> (s? t:f=w177:dbl)
    n117 = feedback-in #4(w177) -> ()
    n118 = Subtract(x=w150, y=w177) -> (x-y=w172:dbl)
    n119 = call "Moving_Avg.vi"("Num_Avg"="Num_Avg", "Numeric in"=w172) -> ("Numeric out"=w171:dbl)  [unwired: 9 in]
    "Yaw" <- w171
    n120 = global write "Global Var.vi" "Yaw"(w171) -> ()
  }
  n121 = while {
    shift-right: [w208] -> _
    shift-left: w1 -> [w208]
    stop <- FALSE stop-if-true
    n122 = call "RIOduino Periodic.vi"() -> ()  [unwired: 12 in]
    n123 = Wait (ms)(milliseconds to wait=u32 100) -> ()  [unwired: 1 out]
  }
  n124 = while {
    shift-right: [w212] -> _
    shift-left: w1 -> [w212]
    stop <- FALSE stop-if-true
    # "Get the value from the compressor \nto see if the system is monitoring the pressure"
    # "Compressor"
    n125 = Unbundle By Name(w212) -> ("Pneumatics.Compressor"=w211:T26)
    n126 = call <vilib>:"WPI_CompressorGetEnableState.vi"("CompressorDevRef"=w211) -> ("Compressor Running"=→"Compressor Running":bool, "Enabled"=→"Compressor Monitoring":bool)  [unwired: 1 in, 8 out]
    n127 = Wait (ms)(milliseconds to wait=u32 100) -> ()  [unwired: 1 out]
  }
